vi "Unpack Gamepad.vi"(11 "JoystickDevRef":T2) -> (0 "Button Array":bool[](array[boolean]), 1 "D-Pad":T1, 2 "Button Cluster":T4, 3 "Axes":T5)   [LabVIEW 2014]
uses:
  <vilib>/Rock Robotics/WPI/Joystick/WPI_JoystickDevRef.ctl
  <vilib>/Rock Robotics/WPI/Joystick/WPI_JoystickDeviceEnum.ctl
  D-Pad.ctl
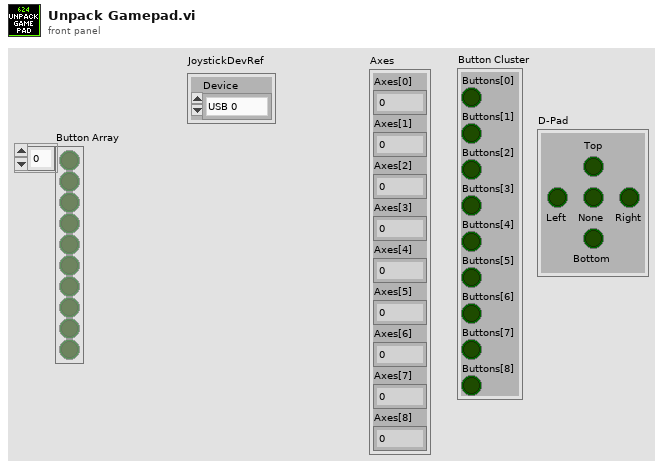
[diagram p1: front panel]
types:
  T1 = typedef "D-Pad.ctl" = cluster{"Top":bool, "Bottom":bool, "None":bool, "Right":bool, "Left":bool}
  T2 = typedef "WPI_JoystickDevRef.ctl" = cluster{"Device":T3}
  T3 = typedef "WPI_JoystickDeviceEnum.ctl" = enum16{"USB 0", "USB 1", "USB 2", "USB 3", "USB 4", "USB 5"}
  T4 = cluster{"Buttons[0]":bool, "Buttons[1]":bool, "Buttons[2]":bool, "Buttons[3]":bool, "Buttons[4]":bool, "Buttons[5]":bool, "Buttons[6]":bool, "Buttons[7]":bool, "Buttons[8]":bool}
  T5 = cluster{"Axes[0]":dbl, "Axes[1]":dbl, "Axes[2]":dbl, "Axes[3]":dbl, "Axes[4]":dbl, "Axes[5]":dbl, "Axes[6]":dbl, "Axes[7]":dbl, "Axes[8]":dbl}
  T6 = cluster{"POVs[0]":i16, "POVs[1]":i16, "POVs[2]":i16, "POVs[3]":i16, "POVs[4]":i16, "POVs[5]":i16, "POVs[6]":i16, "POVs[7]":i16, "POVs[8]":i16}
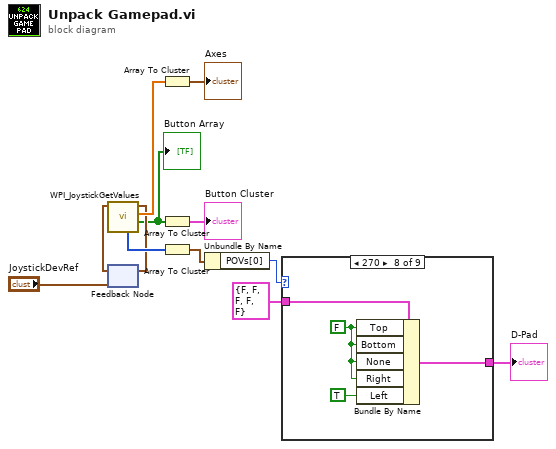
[diagram p0: block diagram]
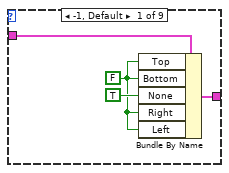
[diagram p2: hidden frame]
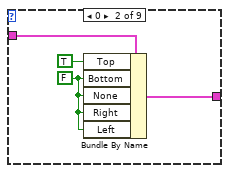
[diagram p3: hidden frame]
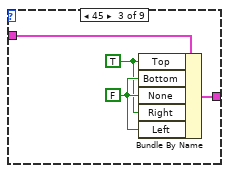
[diagram p4: hidden frame]
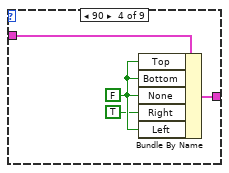
[diagram p5: hidden frame]
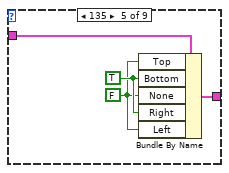
[diagram p6: hidden frame]
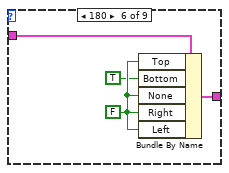
[diagram p7: hidden frame]
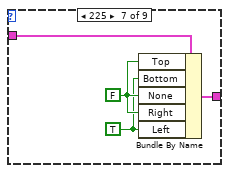
[diagram p8: hidden frame]
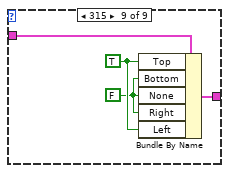
[diagram p9: hidden frame]
diagram:
  n1 = feedback #1("JoystickDevRef") -> (w7:T2)
  n2 = call <vilib>:"WPI_JoystickGetValues.vi"("JoystickDevRef"=w7) -> ("Buttons"=w6:bool[], "Axes"=w12:dbl[], "JoystickDevRef"=w8:T2, "POVs"=w10:i16[])  [unwired: 6 in, 1 out]
  "Button Array" <- w6
  n3 = feedback-in #1(w8) -> ()
  n4 = Array To Cluster(array=w12) -> (cluster=→"Axes":T5)
  n5 = Array To Cluster(array=w6) -> (cluster=→"Button Cluster":T4)
  n6 = Array To Cluster(array=w10) -> (cluster=w4:T6)
  n7 = Unbundle By Name(w4) -> ("POVs[0]"=w3:i16)
  n8 = case shown="270" w3 {
    tunnel: T1 {"Top"=FALSE, "Bottom"=FALSE, "None"=FALSE, "Right"=FALSE, "Left"=FALSE} ("D-Pad") -> [w14 w20 w24 w28 w32 w36 w40 w44 w48]
    tunnel: [w13 w19 w23 w27 w31 w35 w39 w43 w47] -> w1
    frame -1, Default {
      w15 = FALSE
      n9 = Bundle By Name(cluster=w14, "Top"=w15, "Bottom"=w15, "None"=TRUE, "Right"=w15, "Left"=w15) -> (w13:T1)
    }
    frame 0 {
      w17 = FALSE
      n10 = Bundle By Name(cluster=w20, "Top"=TRUE, "Bottom"=w17, "None"=w17, "Right"=w17, "Left"=w17) -> (w19:T1)
    }
    frame 45 {
      w22 = FALSE
      w21 = TRUE
      n11 = Bundle By Name(cluster=w24, "Top"=w21, "Bottom"=w22, "None"=w22, "Right"=w21, "Left"=w22) -> (w23:T1)
    }
    frame 90 {
      w26 = FALSE
      n12 = Bundle By Name(cluster=w28, "Top"=w26, "Bottom"=w26, "None"=w26, "Right"=TRUE, "Left"=w26) -> (w27:T1)
    }
    frame 135 {
      w29 = FALSE
      w30 = TRUE
      n13 = Bundle By Name(cluster=w32, "Top"=w29, "Bottom"=w30, "None"=w29, "Right"=w30, "Left"=w29) -> (w31:T1)
    }
    frame 180 {
      w34 = FALSE
      n14 = Bundle By Name(cluster=w36, "Top"=w34, "Bottom"=TRUE, "None"=w34, "Right"=w34, "Left"=w34) -> (w35:T1)
    }
    frame 225 {
      w38 = FALSE
      w37 = TRUE
      n15 = Bundle By Name(cluster=w40, "Top"=w38, "Bottom"=w37, "None"=w38, "Right"=w38, "Left"=w37) -> (w39:T1)
    }
    frame 270 {
      w41 = FALSE
      n16 = Bundle By Name(cluster=w44, "Top"=w41, "Bottom"=w41, "None"=w41, "Right"=w41, "Left"=TRUE) -> (w43:T1)
    }
    frame 315 {
      w45 = FALSE
      w46 = TRUE
      n17 = Bundle By Name(cluster=w48, "Top"=w46, "Bottom"=w45, "None"=w45, "Right"=w45, "Left"=w46) -> (w47:T1)
    }
  }
  "D-Pad" <- w1
